vi "Main.vi"(10 "DAQ Type":enum16{"Hardware", "Simulation"}(ring), 11 "Module Admin":refnum<class "Delacor_lib_QMH_Module Admin.lvclass">) -> ()   [LabVIEW 2021, in "Calibration.lvlib"]
doc: "This template is based off of the Queued Message Handler design pattern and the Queued Message Handler project template that ships with LabVIEW.\n\nThe main difference is that the queue is private to this module and communication between modules is performed via Broadcast and Request events.\n\nRequest events are wrapped in public API methods and are handled in the Event Handling Loop (EHL) of this VI. Any module can register for Broadcast events sent by this module. The EHL generates messages based on user interface actions.\n\nThe Message Handling Loop (MHL) processes messages generated by the EHL, or by other messages. The messages are string values, so new messages can be added easily to the Message Cases case structure in the MHL. Each message cluster can also provide an optional value for Message Data, which is a variant that can be converted to whatever message-specific data is required.\n_____\nBased on DQMH Project Template 6.1.0.94."
uses:
  Calibration.lvlib
  <vilib>/Delacor/Delacor QMH/Libraries/Module Admin_class/Delacor_lib_QMH_Module Admin.lvclass
  Module Data--cluster.ctl
  <vilib>/Delacor/Delacor QMH/Libraries/Message Queue_class/Delacor_lib_QMH_Message Queue.lvclass/Delacor_lib_QMH_Message Queue.ctl
  Stop Argument--cluster.ctl
  <vilib>/Delacor/Delacor QMH/Libraries/Module Admin_class/Delacor_lib_QMH_Module Admin.lvclass/Delacor_lib_QMH_Module Admin.ctl
  REQ Initialize Argument--cluster.ctl
  REQ Calibration Details Argument--cluster.ctl
  REQ Calibration Details (Reply Payload)--cluster.ctl
  REQ Update Calibration Argument--cluster.ctl
  REQ Check Calibration Argument--cluster.ctl
  REQ Check Calibration (Reply Payload)--cluster.ctl
  <vilib>/Utility/miscctls.llb/LVPointTypeDef.ctl
  Calibration Command.ctl
  <vilib>/Delacor/Delacor QMH/Libraries/Message Queue_class/Delacor_lib_QMH_Enqueue Message (Single).vi
  <vilib>/Delacor/Delacor QMH/Libraries/Module Admin_class/Delacor_lib_QMH_Get External Launch.vi
  <vilib>/Utility/error.llb/Error Cluster From Error Code.vi
  <vilib>/ErrorRing/Error Ring.xnode
  <vilib>/Delacor/Delacor QMH/Libraries/Message Queue_class/Delacor_lib_QMH_Message Queue.lvclass
panel:
  out "error out":errorcluster
  out "Status":string
  in  "Simulate MHL Error":bool
  in  "Simulate EHL Error":bool
  # "Other QMH Modules communicate with this Module via its Public API (wrappers for its Request Events).\n\nThis Module communicates with other Modules via its Broadcast Events.\nAny module that wants to get these messages, just registers for this module's Broadcast events."
  # "This template is for the Delacor Modified Queued Message Handler design pattern.\n\nSee the block diagram for more information on how to use this template."
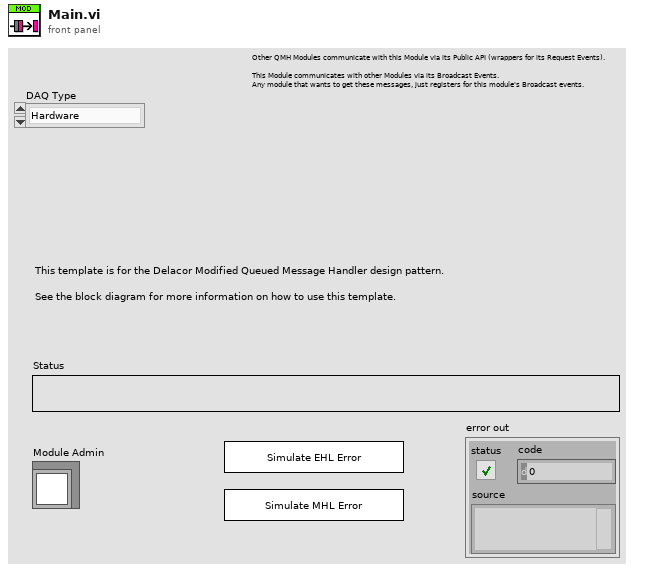
[diagram p1: front panel]
types:
  T1 = typedef "Calibration.lvlib/Request Events--cluster.ctl" = cluster{"Stop Module":refnum<user-event>, "Show Panel":refnum<user-event>, "Hide Panel":refnum<user-event>, "Get Module Execution Status":refnum<user-event>, "Show Diagram":refnum<user-event>, "REQ Initialize":refnum<user-event>, "REQ Calibration Details":refnum<user-event>, "REQ Update Calibration":refnum<user-event>, "REQ Check Calibration":refnum<user-event>}
  T2 = typedef "Calibration.lvlib/Module Data--cluster.ctl" = cluster{"Status":string}
  T3 = enum32{"invalid lock state", "Not Locked", "Locked (No Password)", "Password-protected"}
  T4 = typedef "Calibration.lvlib/Stop Argument--cluster.ctl" = cluster{"Origin":string, "Exit via Stop Module Req?":bool, "Wait for Module to stop?":bool}
  T5 = typedef "Calibration.lvlib/REQ Initialize Argument--cluster.ctl" = cluster{"Boolean":bool}
  T6 = typedef "Calibration.lvlib/REQ Calibration Details Argument--cluster.ctl" = cluster{"Wait Notifier":refnum<notifier>, "wait for reply":bool}
  T7 = typedef "Calibration.lvlib/REQ Update Calibration Argument--cluster.ctl" = cluster{"Calibration Details In":string[][]}
  T8 = typedef "Calibration.lvlib/REQ Check Calibration Argument--cluster.ctl" = cluster{"Wait Notifier":refnum<notifier>, "wait for reply":bool}
  T9 = typedef "LVPointTypeDef.ctl" = cluster{"Horizontal":i16, "Vertical":i16}
  T10 = enum32{"Invalid", "Standard", "Closed", "Hidden", "Minimized", "Maximized"}
  T11 = typedef "Calibration.lvlib/Calibration Command.ctl" = enum16{"Init", "Read", "Write", "Check Calibration", "Close"}
  T12 = typedef "Calibration.lvlib/REQ Calibration Details (Reply Payload)--cluster.ctl" = cluster{"Calibration Details":string[][], "error":errorcluster}
  T13 = typedef "Calibration.lvlib/REQ Check Calibration (Reply Payload)--cluster.ctl" = cluster{"Calibration Due Msg":string[], "error":errorcluster}
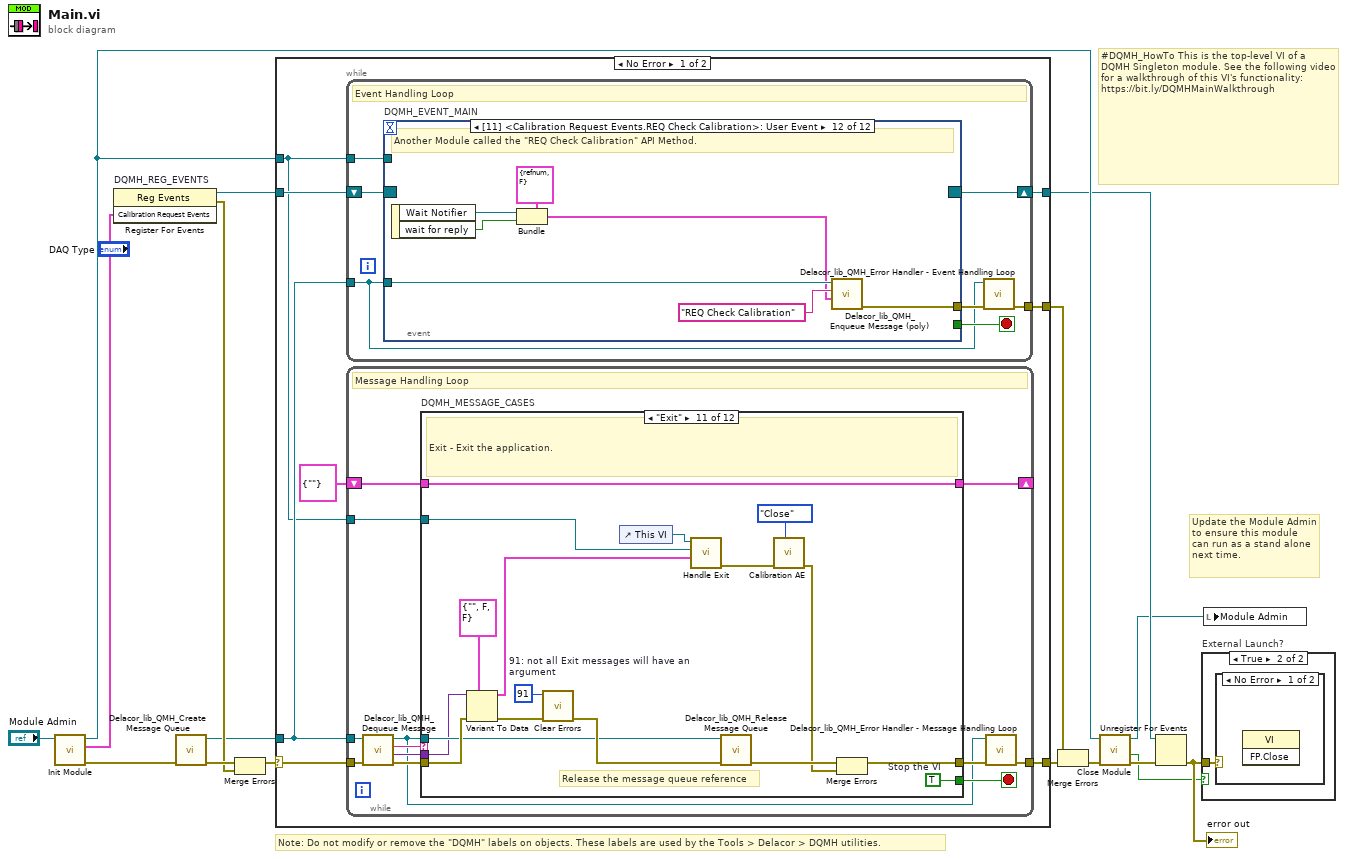
[diagram p0: block diagram]
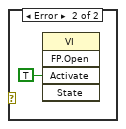
[diagram p3: hidden frame]
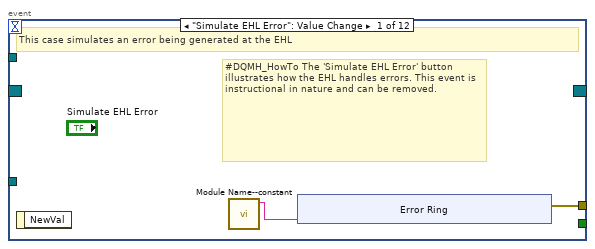
[diagram p4: hidden frame]
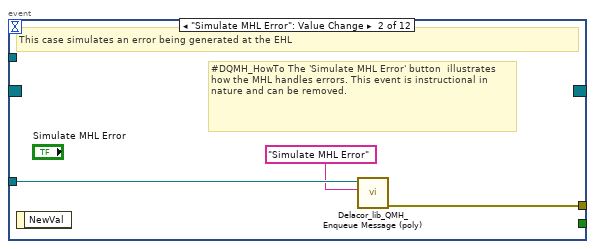
[diagram p5: hidden frame]
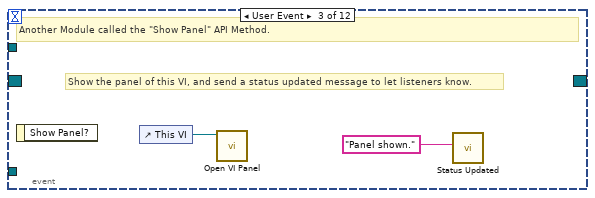
[diagram p6: hidden frame]
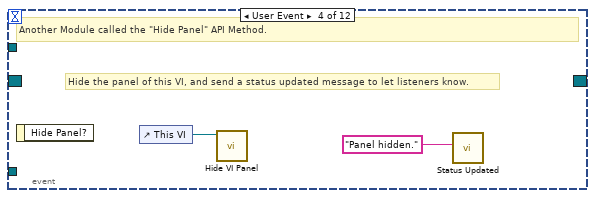
[diagram p7: hidden frame]
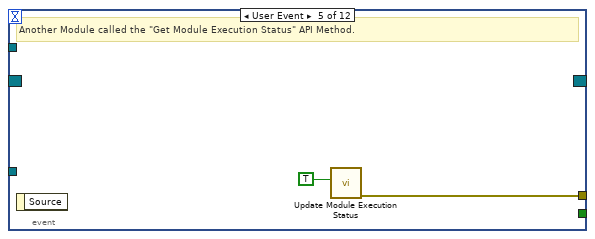
[diagram p8: hidden frame]
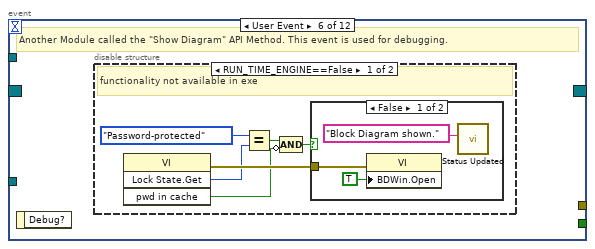
[diagram p9: hidden frame]
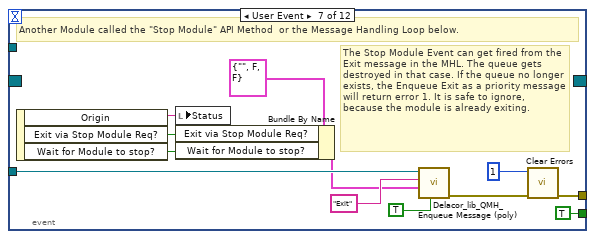
[diagram p12: hidden frame]
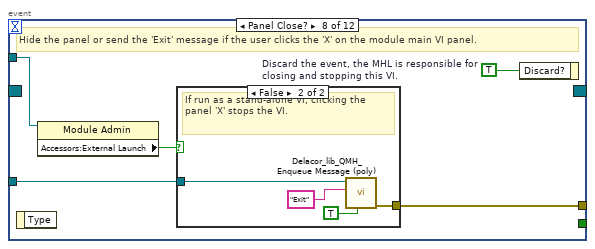
[diagram p13: hidden frame]
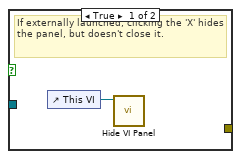
[diagram p14: hidden frame]
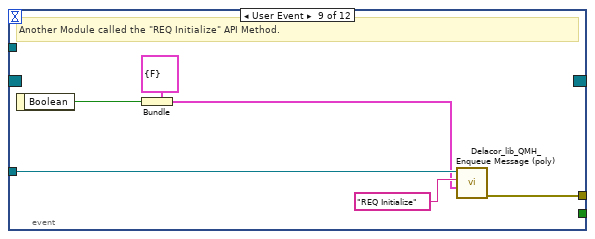
[diagram p15: hidden frame]
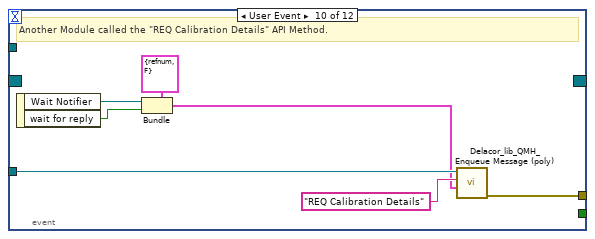
[diagram p16: hidden frame]
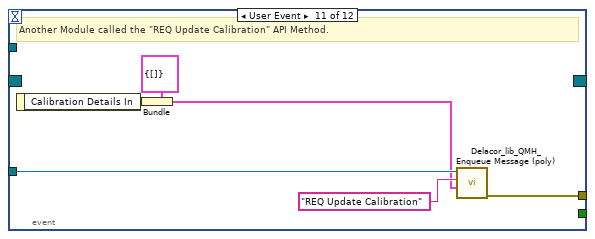
[diagram p17: hidden frame]
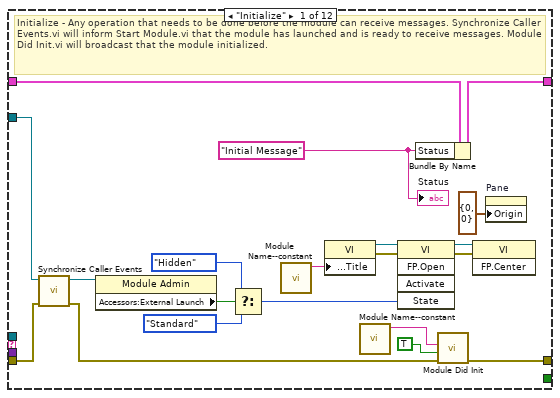
[diagram p18: hidden frame]
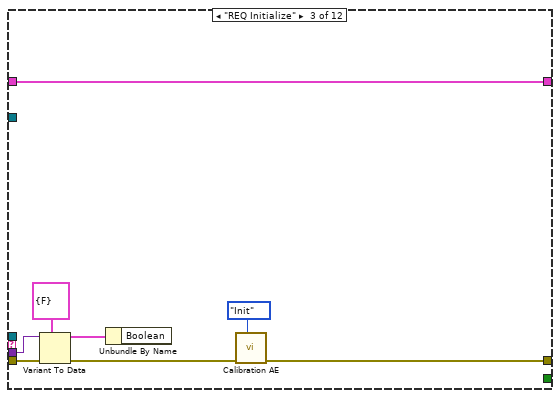
[diagram p20: hidden frame]
diagram:
  # "#DQMH_HowTo This is the top-level VI of a DQMH Singleton module. See the following video for a walkthrough of this VI's functionality: https://bit.ly/DQMHMainWalkthrough"
  # "Note: Do not modify or remove the \"DQMH\" labels on objects. These labels are used by the Tools > Delacor > DQMH utilities."
  # "Update the Module Admin to ensure this module can run as a stand alone next time."
  n1 = call "Init Module.vi"("Singleton Module Admin in"="Module Admin") -> ("error out"=w16:errorcluster, "Calibration Request Events"=w5:T1, "Singleton Module Admin out"=w8:refnum<class "Delacor_lib_QMH_Module Admin.lvclass">)  [unwired: 8 in]
  n2 = register-events "DQMH_REG_EVENTS"(w5) -> (reference out=w6:refnum<event-registration>, error out=w9:errorcluster)  [unwired: 2 in]
  n3 = call <vilib>:"Delacor_lib_QMH_Create Message Queue.vi"("error in"=w16) -> ("error out"=w11:errorcluster, "Message Queue"=w4:refnum<class "Delacor_lib_QMH_Message Queue.lvclass">)  [unwired: 9 in]
  n4 = Merge Errors(w11, w9) -> (w10:errorcluster)
  n5 = case shown="No Error" w10 {
    selector: w10 -> [w23 w255]
    tunnel: [w25 w254] -> w17
    tunnel: [w22 w260] -> w7
    tunnel: w6 -> [w20 w260]
    tunnel: w4 -> [w19 w253]
    tunnel: [w24 _] -> w14
    tunnel: w8 -> [w18 w256]
    frame No Error {
      n6 = while {
        tunnel: w19 -> [w26]
        shift-right: [w29] -> w22
        shift-left: w20 -> [w30]
        tunnel: [w31] -> w24
        tunnel: w18 -> [w27]
        stop <- w28 stop-if-true
        # "Event Handling Loop"
        n7 = event "DQMH_EVENT_MAIN" shown="[11] <Calibration Request Events.REQ Check Calibration>: User Event" {
          selector: w30 -> [_ _ _ _ _ _ _ _ _ _ _ _]
          dyn-events: [_ _ _ _ _ _ _ _ _ _ _ _] -> w29
          timeout: _ -> [_ _ _ _ _ _ _ _ _ _ _ _]
          tunnel: [_ _ _ _ _ _ TRUE ("Discard?") _ _ _ _ _] -> w28
          tunnel: w26 -> [_ w43 _ _ _ _ w67 w74 w87 w94 w100 w107]
          tunnel: [w34 w44 _ _ w50 _ w70 w76 w82 w88 w95 w101] -> w32
          tunnel: w27 -> [_ _ _ _ _ _ _ w73 _ _ _ _]
          event "Simulate EHL Error": Value Change {
            # "#DQMH_HowTo The 'Simulate EHL Error' button  illustrates how the EHL handles errors. This event is instructional in nature and can be removed."
            # "This case simulates an error being generated at the EHL"
            n8 = event-data() -> ()  [unwired: 1 in, 1 out]
            n9 = call "Module Name--constant.vi"() -> ("Module Name"=w33:string)  [unwired: 11 in]
            n10 = xnode "Error Ring"("parameter 0"=w33) -> ("error out"=w34:errorcluster)
          }
          event "Simulate MHL Error": Value Change {
            # "#DQMH_HowTo The 'Simulate MHL Error' button  illustrates how the MHL handles errors. This event is instructional in nature and can be removed."
            # "This case simulates an error being generated at the EHL"
            n11 = event-data() -> ()  [unwired: 1 in, 1 out]
            n12 = call-poly <vilib>:"Delacor_lib_QMH_Enqueue Message (poly).vi"("Message"="Simulate MHL Error", "Message Queue in"=w43) -> ("error out"=w44:errorcluster)  [unwired: 8 in, 1 out]
          }
          event User Event {
            # "Show the panel of this VI, and send a status updated message to let listeners know."
            # "Another Module called the \"Show Panel\" API Method."
            n13 = event-data() -> ()  [unwired: 1 in, 1 out]
            n14 = control-ref of="This VI"() -> (w46:refnum<vi>)
            n15 = call "Open VI Panel.vi"("VI"=w46) -> ()  [unwired: 10 in, 1 out]
            n16 = call "Status Updated.vi"("Status"="Panel shown." ("format string")) -> ()  [unwired: 10 in, 1 out]
          }
          event User Event {
            # "Hide the panel of this VI, and send a status updated message to let listeners know."
            # "Another Module called the \"Hide Panel\" API Method."
            n17 = event-data() -> ()  [unwired: 1 in, 1 out]
            n18 = control-ref of="This VI"() -> (w48:refnum<vi>)
            n19 = call "Hide VI Panel.vi"("VI"=w48) -> ()  [unwired: 10 in, 1 out]
            n20 = call "Status Updated.vi"("Status"="Panel hidden." ("format string")) -> ()  [unwired: 10 in, 1 out]
          }
          event User Event {
            # "Another Module called the \"Get Module Execution Status\" API Method."
            n21 = event-data() -> ()  [unwired: 1 in, 1 out]
            n22 = call "Update Module Execution Status.vi"("Running?"=TRUE) -> ("error out"=w50:errorcluster)  [unwired: 10 in]
          }
          event User Event {
            # "Another Module called the \"Show Diagram\" API Method. This event is used for debugging."
            n23 = event-data() -> ()  [unwired: 1 in, 1 out]
            n24 = disable-structure shown="RUN_TIME_ENGINE==False" {
              frame condition #0 (active) {
                # "functionality not available in exe"
                n25 = invoke class="VI" method="Lock State.Get"() -> (error out=w56:errorcluster, "Get Lock State"=w55:T3, "pwd in cache"=w52:bool)  [unwired: 4 in, 1 out]
                n26 = Equal?(x=T3."Password-protected", y=w55) -> (x = y?=w53:bool)
                n27 = Compound Arithmetic op=AND(w53, invert w52) -> (w51:bool)
                n28 = case shown="False" w51 {
                  tunnel: w56 -> [w59 _]
                  frame False {
                    n29 = property class="VI"(error in=w59, "BDWin.Open"=TRUE ("Block Diagram Window:Open")) -> ()  [unwired: 1 in, 2 out]
                    n30 = call "Status Updated.vi"("Status"="Block Diagram shown." ("format string")) -> ()  [unwired: 10 in, 1 out]
                  }
                  frame True {
                    # "Password-protected VI, and the password is not in the cache. Do not show the diagram."
                  }
                }
              }
              frame condition #1 {
              }
            }
          }
          event User Event {
            # "The Stop Module Event can get fired from the Exit message in the MHL. The queue gets destroyed in that case. If the queue no longer exists, the Enqueue Exit as a priority message will return error 1. It is safe to ignore, because the module is already exiting."
            # "Another Module called the \"Stop Module\" API Method  or the Message Handling Loop below."
            n31 = event-data() -> ("Origin"=w66:string, "Exit via Stop Module Req?"=w62:bool, "Wait for Module to stop?"=w61:bool)  [unwired: 1 in]
            n32 = local write "Status"(w66) -> ()
            n33 = Bundle By Name(cluster=T4 {"Origin"="", "Exit via Stop Module Req?"=FALSE, "Wait for Module to stop?"=FALSE} ("Stop Argument"), "Exit via Stop Module Req?"=w62, "Wait for Module to stop?"=w61) -> (w60:T4)
            n34 = call-poly <vilib>:"Delacor_lib_QMH_Enqueue Message (poly).vi"("Priority Message? (F)"=TRUE, "Message Data"=w60, "Message"="Exit", "Message Queue in"=w67) -> ("error out"=w71:errorcluster)  [unwired: 6 in, 1 out]
            n35 = call <vilib>:"Clear Errors.vi"("error in (no error)"=w71, "specific error code to clear (0: all)"=1) -> ("error out"=w70:errorcluster)  [unwired: 4 in, 1 out]
          }
          event Panel Close? {
            w75 = TRUE  # Discard the event, the MHL is responsible for closing and stopping this VI.
            # "Hide the panel or send the 'Exit' message if the user clicks the 'X' on the module main VI panel."
            n36 = event-data() -> ()  [unwired: 1 in, 1 out]
            n37 = property class="Module Admin"(reference=w73) -> ("Accessors:External Launch"=w72:bool)  [unwired: 1 in, 2 out]
            n38 = case shown="False" w72 {
              tunnel: w74 -> [_ w80]
              tunnel: [_ w81] -> w76
              frame True {
                # "If externally launched, clicking the 'X' hides the panel, but doesn't close it."
                n39 = control-ref of="This VI"() -> (w77:refnum<vi>)
                n40 = call "Hide VI Panel.vi"("VI"=w77) -> ()  [unwired: 10 in, 1 out]
              }
              frame False {
                # "If run as a stand-alone VI, clicking the panel 'X' stops the VI."
                n41 = call-poly <vilib>:"Delacor_lib_QMH_Enqueue Message (poly).vi"("Priority Message? (F)"=TRUE, "Message"="Exit", "Message Queue in"=w80) -> ("error out"=w81:errorcluster)  [unwired: 7 in, 1 out]
              }
            }
            n42 = event-data("Discard?"=w75) -> ()  [unwired: 1 in, 1 out]
          }
          event User Event {
            # "Another Module called the \"REQ Initialize\" API Method."
            n43 = event-data() -> ("Boolean"=w83:bool)  [unwired: 1 in]
            n44 = Bundle(cluster=T5 {"Boolean"=FALSE} ("REQ Initialize Argument"), "Boolean"=w83) -> (w84:T5)
            n45 = call-poly <vilib>:"Delacor_lib_QMH_Enqueue Message (poly).vi"("Message Data"=w84, "Message"="REQ Initialize", "Message Queue in"=w87) -> ("error out"=w82:errorcluster)  [unwired: 7 in, 1 out]
          }
          event User Event {
            # "Another Module called the \"REQ Calibration Details\" API Method."
            n46 = event-data() -> ("Wait Notifier"=w90:refnum<notifier>, "wait for reply"=w89:bool)  [unwired: 1 in]
            n47 = Bundle(cluster=T6 {"Wait Notifier"=refnum, "wait for reply"=FALSE} ("REQ Calibration Details Argument"), "Wait Notifier"=w90, "wait for reply"=w89) -> (w91:T6)
            n48 = call-poly <vilib>:"Delacor_lib_QMH_Enqueue Message (poly).vi"("Message Data"=w91, "Message"="REQ Calibration Details", "Message Queue in"=w94) -> ("error out"=w88:errorcluster)  [unwired: 7 in, 1 out]
          }
          event User Event {
            # "Another Module called the \"REQ Update Calibration\" API Method."
            n49 = event-data() -> ("Calibration Details In"=w96:string[][])  [unwired: 1 in]
            n50 = Bundle(cluster=T7 {"Calibration Details In"=[]} ("REQ Update Calibration Argument"), "Calibration Details In"=w96) -> (w97:T7)
            n51 = call-poly <vilib>:"Delacor_lib_QMH_Enqueue Message (poly).vi"("Message Data"=w97, "Message"="REQ Update Calibration", "Message Queue in"=w100) -> ("error out"=w95:errorcluster)  [unwired: 7 in, 1 out]
          }
          event User Event {
            # "Another Module called the \"REQ Check Calibration\" API Method."
            n52 = event-data() -> ("Wait Notifier"=w103:refnum<notifier>, "wait for reply"=w102:bool)  [unwired: 1 in]
            n53 = Bundle(cluster=T8 {"Wait Notifier"=refnum, "wait for reply"=FALSE} ("REQ Check Calibration Argument"), "Wait Notifier"=w103, "wait for reply"=w102) -> (w104:T8)
            n54 = call-poly <vilib>:"Delacor_lib_QMH_Enqueue Message (poly).vi"("Message Data"=w104, "Message"="REQ Check Calibration", "Message Queue in"=w107) -> ("error out"=w101:errorcluster)  [unwired: 7 in, 1 out]
          }
        }
        n55 = call-dynamic "Delacor_lib_QMH_Error Handler - Event Handling Loop.vi"("error in"=w32, "Message Queue in"=w26) -> ("dup error in"=w31:errorcluster)  [unwired: 8 in, 1 out]
      }
      n56 = while {
        tunnel: w19 -> [w110]
        shift-right: [w114] -> _
        shift-left: T2 {"Status"=""} ("Data Cluster") -> [w115]
        tunnel: w23 -> [w118]
        tunnel: [w116] -> w25
        tunnel: w18 -> [w108]
        stop <- w113 stop-if-true
        # "Message Handling Loop"
        n57 = call-dynamic "Delacor_lib_QMH_Dequeue Message.vi"("error in"=w118, "Message Queue in"=w110) -> ("error out"=w117:errorcluster, "Message Data"=w111:variant, "Message"=w112:string, "Message Queue out"=w109:refnum<class "Delacor_lib_QMH_Message Queue.lvclass">)  [unwired: 6 in]
        n58 = case "DQMH_MESSAGE_CASES" shown="\"Exit\"" w112 {
          selector: w112 -> [_ _ _ _ _ _ _ _ _ _ _ w240]
          tunnel: w109 -> [_ _ _ _ _ _ _ _ _ w208 w233 _]
          tunnel: w117 -> [w137 w141 w149 w162 w173 w186 w191 w193 w198 w215 w238 w242]
          tunnel: [w135 w141 w143 w152 w166 w175 w190 w193 w197 w211 w235 w243] -> w119
          tunnel: w115 -> [w126 w140 w148 w161 w172 w185 w189 w192 w195 w210 w232 w241]
          tunnel: [w125 w140 w148 w161 w172 w185 w189 w192 w195 w210 w232 w241] -> w114
          tunnel: [_ _ _ _ _ _ _ _ _ _ w231 _] -> w113
          tunnel: w111 -> [_ _ w147 w160 w171 w184 _ _ _ w209 w230 _]
          tunnel: w108 -> [w127 _ _ _ _ _ _ _ _ w207 w225 _]
          frame "Initialize" {
            w121 = "Initial Message" ("Initial Message")
            # "Initialize - Any operation that needs to be done before the module can receive messages. Synchronize Caller Events.vi will inform Start Module.vi that the module has launched and is ready to receive messages. Module Did Init.vi will broadcast that the module initialized."
            n59 = call "Synchronize Caller Events.vi"("error in (no error)"=w137, "Singleton Module Admin in"=w127) -> ("error out"=w136:errorcluster, "Singleton Module Admin out"=w122:refnum<class "Delacor_lib_QMH_Module Admin.lvclass">)  [unwired: 8 in]
            n60 = property class="Module Admin"(reference=w122) -> ("Accessors:External Launch"=w131:bool)  [unwired: 1 in, 2 out]
            n61 = Select(t=T10."Hidden" ("State"), s=w131, f=T10."Standard" ("State")) -> (s? t:f=w128:T10)
            n62 = call "Module Name--constant.vi"() -> ("Module Name"=w134:string)  [unwired: 11 in]
            n63 = property class="VI"("Front Panel.Title"=w134) -> (reference out=w133:refnum<vi>, error out=w139:errorcluster)  [unwired: 2 in]
            n64 = call "Module Name--constant.vi"() -> ("Module Name"=w123:string)  [unwired: 11 in]
            n65 = invoke class="VI" method="FP.Open"(reference=w133, error in=w139, "State"=w128) -> (reference out=w132:refnum<vi>, error out=w138:errorcluster)  [unwired: 2 in, 3 out]
            n66 = Bundle By Name(cluster=w126, "Status"=w121) -> (w125:T2)
            n67 = call "Module Did Init.vi"("error in (no error)"=w136, "Initialized?"=TRUE, "Origin"=w123) -> ("error out"=w135:errorcluster)  [unwired: 8 in]
            n68 = invoke class="VI" method="FP.Center"(reference=w132, error in=w138) -> ()  [unwired: 1 in, 3 out]
            n69 = property on="Pane" class="Pane"("Origin"=T9 {"Horizontal"=0, "Vertical"=0}) -> ()  [unwired: 2 in, 2 out]
            "Status" <- w121
          }
          frame "---Module Specific---" {
            # "Separator -- The following cases handle messages specific to this Module."
          }
          frame "REQ Initialize" {
            n70 = Variant To Data(error in=w149, type=T5 {"Boolean"=FALSE} ("REQ Initialize Argument"), Variant=w147) -> (data=w145:T5, error out=w144:errorcluster)
            n71 = Unbundle By Name(w145) -> ()  [unwired: 1 out]
            n72 = call "Calibration AE.vi"("Command"=Calibration_Command."Init", "error in (no error)"=w144) -> ("error out"=w143:errorcluster)  [unwired: 7 in, 2 out]
          }
          frame "REQ Calibration Details" {
            n73 = Variant To Data(error in=w162, type=T6 {"Wait Notifier"=refnum, "wait for reply"=FALSE} ("REQ Calibration Details Argument"), Variant=w160) -> (data=w158:T6, error out=w153:errorcluster)
            n74 = Unbundle By Name(w158) -> ("Wait Notifier"=w157:refnum<notifier>, "wait for reply"=w156:bool)
            n75 = call "Calibration AE.vi"("Command"=Calibration_Command."Read", "error in (no error)"=w153) -> ("error out"=w152:errorcluster, "Inst Details Out"=w151:string[][])  [unwired: 7 in, 1 out]
            n76 = Bundle By Name(cluster=T12 {"Calibration Details"=[], "error"={"status"=FALSE, "code"=0, "source"=""}} ("REQ Calibration Details (Reply Payload)"), "Calibration Details"=w151) -> (w155:T12)
            n77 = case shown="True" w156 {
              tunnel: w157 -> [_ w164]
              tunnel: w155 -> [_ w163]
              frame False {
              }
              frame True {
                n78 = Send Notification(notification=w163, notifier=w164) -> ()  [unwired: 1 in, 2 out]
              }
            }
          }
          frame "REQ Update Calibration" {
            n79 = Variant To Data(error in=w173, type=T7 {"Calibration Details In"=[]} ("REQ Update Calibration Argument"), Variant=w171) -> (data=w169:T7, error out=w168:errorcluster)
            n80 = Unbundle By Name(w169) -> ("Calibration Details In"=w167:string[][])
            n81 = call "Calibration AE.vi"("Command"=Calibration_Command."Write", "error in (no error)"=w168, "Inst Details In"=w167) -> ("error out"=w166:errorcluster)  [unwired: 6 in, 2 out]
          }
          frame "REQ Check Calibration" {
            n82 = Variant To Data(error in=w186, type=T8 {"Wait Notifier"=refnum, "wait for reply"=FALSE} ("REQ Check Calibration Argument"), Variant=w184) -> (data=w182:T8, error out=w176:errorcluster)
            n83 = Unbundle By Name(w182) -> ("Wait Notifier"=w181:refnum<notifier>, "wait for reply"=w180:bool)
            n84 = call "Calibration AE.vi"("Command"=Calibration_Command."Check Calibration", "error in (no error)"=w176) -> ("error out"=w175:errorcluster, "Calibration Due Msg?"=w174:string[])  [unwired: 7 in, 1 out]
            n85 = Bundle By Name(cluster=T13 {"Calibration Due Msg"=[], "error"={"status"=FALSE, "code"=0, "source"=""}} ("REQ Check Calibration (Reply Payload)"), "Calibration Due Msg"=w174) -> (w179:T13)
            n86 = case shown="True" w180 {
              tunnel: w181 -> [_ w188]
              tunnel: w179 -> [_ w187]
              frame False {
              }
              frame True {
                n87 = Send Notification(notification=w187, notifier=w188) -> ()  [unwired: 1 in, 2 out]
              }
            }
          }
          frame "---Copy This Frame---" {
            # "Duplicate this frame when creating new messages.  Change this comment in the duplicated frame to describe this message."
            n88 = Merge Errors(w191) -> (w190:errorcluster)
          }
          frame "---Exit and Error Handling---" {
            # "Separator - The following cases handle errors and exit messages."
          }
          frame "Simulate MHL Error" {
            # "#DQMH_HowTo The 'Simulate MHL Error' button  illustrates how the MHL handles errors. This event is instructional in nature and can be removed."
            # "Simulate an error occurring at the MHL"
            n89 = call "Module Name--constant.vi"() -> ("Module Name"=w194:string)  [unwired: 11 in]
            n90 = xnode "Error Ring"("parameter 0"=w194) -> ("error out"=w196:errorcluster)
            n91 = Merge Errors(w198, w196) -> (w197:errorcluster)
          }
          frame "Error" {
            # "#CodeRecommended - If you ever change the name of this \"Error\" message, you'll need to update the name in the Check Loop Error.vi as well."
            # "#CodeRecommended - If the module is running in standalone mode (External Launch = FALSE), this code will pop up an error dialog and call the 'Exit' message if an error occurs. Add more fine-grained error handling here."
            # "Error - Check the error message data and respond accordingly. This message is sent by the \"Error Handler\" VIs at the end of each loop in this application."
            n92 = property class="Module Admin"(reference=w207) -> ("Accessors:External Launch"=w206:bool)  [unwired: 1 in, 2 out]
            n93 = Variant To Data(error in=w215, type=errorcluster {"status"=FALSE, "code"=0, "source"=""} ("error constant"), Variant=w209) -> (data=w216:errorcluster, error out=w213:errorcluster)
            n94 = call "Error Reported.vi"("Error"=w216) -> ()  [unwired: 10 in, 1 out]
            n95 = case shown="False" w206 {
              tunnel: [w221 _] -> w212
              tunnel: w208 -> [w219 _]
              tunnel: w216 -> [w220 _]
              frame False {
                # "If the module is running standalone, then pop up an error dialog and call the \"Exit\" message."
                n96 = call <vilib>:"Simple Error Handler.vi"("error in (no error)"=w220) -> ()  [unwired: 4 in, 5 out]
                n97 = call-poly <vilib>:"Delacor_lib_QMH_Enqueue Message (poly).vi"("Priority Message? (F)"=TRUE, "Message"="Exit", "Message Queue in"=w219) -> ("error out"=w221:errorcluster)  [unwired: 7 in, 1 out]
              }
              frame True {
                # "If the module was launched externally, calling the Error Reported broadcast VI is the only action performed by the \"Error\" message. The module's caller can then process the error appropriately."
              }
            }
            n98 = Merge Errors(w213, w212) -> (w211:errorcluster)
            n99 = local write "error out"(w211) -> ()
          }
          frame "Exit" {
            w229 = 91  # 91: not all Exit messages will have an argument
            w231 = TRUE  # Stop the VI
            # "Release the message queue reference"
            # "Exit - Exit the application."
            n100 = Variant To Data(error in=w238, type=T4 {"Origin"="", "Exit via Stop Module Req?"=FALSE, "Wait for Module to stop?"=FALSE} ("Stop Argument"), Variant=w230) -> (data=w227:T4, error out=w234:errorcluster)
            n101 = call <vilib>:"Clear Errors.vi"("error in (no error)"=w234, "specific error code to clear (0: all)"=w229) -> ("error out"=w237:errorcluster)  [unwired: 4 in, 1 out]
            n102 = control-ref of="This VI"() -> (w226:refnum<vi>)
            n103 = call "Handle Exit.vi"("Stop Argument"=w227, "Admin in"=w225, "VI reference"=w226) -> ("error out"=w223:errorcluster)  [unwired: 7 in, 1 out]
            n104 = call-dynamic "Delacor_lib_QMH_Release Message Queue.vi"("error in"=w237, "Message Queue"=w233) -> ("error out"=w236:errorcluster)  [unwired: 9 in]
            n105 = call "Calibration AE.vi"("Command"=Calibration_Command."Close", "error in (no error)"=w223) -> ("error out"=w222:errorcluster)  [unwired: 7 in, 2 out]
            n106 = Merge Errors(w236, w222) -> (w235:errorcluster)
          }
          frame Default {
            # "'Default' case only runs if there is a message that isn't defined in any of the other cases.  Output a programming error."
            n107 = call "Module Name--constant.vi"() -> ("Module Name"=w239:string)  [unwired: 11 in]
            n108 = xnode "Error Ring"("parameter 0"=w240, "parameter 1"=w239) -> ("error out"=w244:errorcluster)
            n109 = Merge Errors(w242, w244) -> (w243:errorcluster)
          }
        }
        n110 = call-dynamic "Delacor_lib_QMH_Error Handler - Message Handling Loop.vi"("error in"=w119, "Message Queue in"=w109) -> ("dup error in"=w116:errorcluster)  [unwired: 8 in, 1 out]
      }
    }
    frame Error {
      # "Synchronize Caller Events.vi will inform Start Module.vi that the module has launched and will let the code calling Start Module.vi register for broadcasts and would permit the caller receive the broadcast that an error occurred at launch time."
      n111 = call-dynamic "Delacor_lib_QMH_Release Message Queue.vi"("error in"=w255, "Message Queue"=w253) -> ("error out"=w254:errorcluster)  [unwired: 9 in]
      n112 = call "Synchronize Caller Events.vi"("Singleton Module Admin in"=w256) -> ("error out"=w261:errorcluster)  [unwired: 9 in, 1 out]
      n113 = call "Module Name--constant.vi"() -> ("Module Name"=w259:string)  [unwired: 11 in]
      n114 = Format Into String(format string="An error occurred during initialization. %s is no longer running.", w259) -> (resulting string=w257:string)  [unwired: 2 in, 1 out]
      n115 = Merge Errors(w254, w261) -> (w262:errorcluster)
      n116 = call "Error Reported.vi"("Additional Information"=w257, "Error"=w262) -> ()  [unwired: 9 in, 1 out]
    }
  }
  n117 = Merge Errors(w14, w17) -> (w13:errorcluster)
  n118 = call "Close Module.vi"("error in (no error)"=w13, "Module Admin in"=w8) -> ("error out"=w15:errorcluster, "External Launch"=w1:bool, "Module Admin out"=w2:refnum<class "Delacor_lib_QMH_Module Admin.lvclass">)  [unwired: 7 in]
  n119 = Unregister For Events(event registration refnum=w7, error in=w15) -> (error out=w12:errorcluster)
  "error out" <- w12
  n120 = case "External Launch?" shown="True" w1 {
    tunnel: w12 -> [_ w263]
    frame False {
    }
    frame True {
      n121 = case shown="No Error" w263 {
        frame No Error {
          n122 = invoke class="VI" method="FP.Close"() -> ()  [unwired: 3 in, 3 out]
        }
        frame Error {
          n123 = invoke class="VI" method="FP.Open"("Activate"=TRUE ("Activate?")) -> ()  [unwired: 4 in, 5 out]
        }
      }
    }
  }
  n124 = local write "Module Admin"(w2) -> ()
